vi "Save Date Yields.vi"(8 "error in (no error)":errorcluster, 10 "Cluster":T1, 11 "Master in":refnum<class "Master.lvclass">) -> (0 "error out":errorcluster, 3 "Master out":refnum<class "Master.lvclass">)   [LabVIEW 2014, in "Master.lvclass"]
uses:
  Master/Master.lvclass
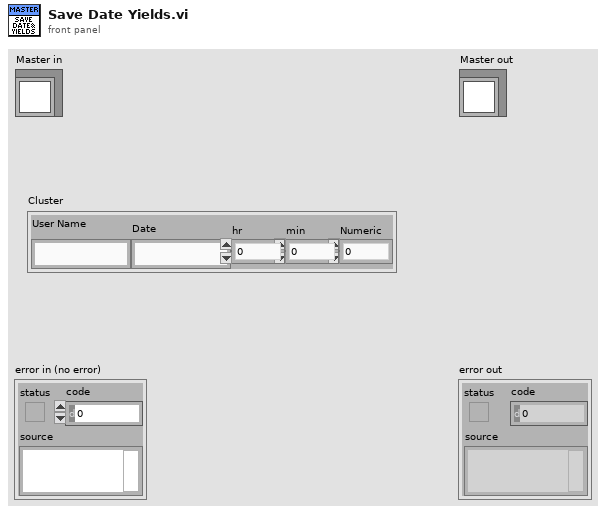
[diagram p1: front panel]
types:
  T1 = cluster{"User Name":string, "Date":string, "Numeric":dbl, "min":dbl, "hr":dbl}
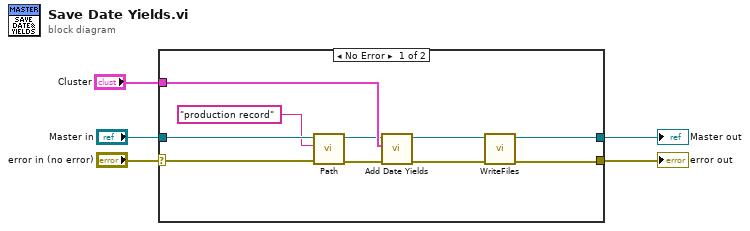
[diagram p0: block diagram]
diagram:
  n1 = case shown="No Error" "error in (no error)" {
    selector: "error in (no error)" -> [w14 w17]
    tunnel: [w11 w17] -> w4
    tunnel: [w12 w16] -> w2
    tunnel: "Master in" -> [w15 w16]
    tunnel: "Cluster" -> [w10 _]
    frame No Error {
      n2 = call-dynamic "Path.vi"("error in (no error)"=w14, "pathname"="production record", "Master in"=w15) -> ("error out"=w8:errorcluster, "Master out"=w9:refnum<class "Master.lvclass">)  [unwired: 7 in]
      n3 = call-dynamic "Add Date Yields.vi"("error in (no error)"=w8, "Cluster"=w10, "Master in"=w9) -> ("error out"=w6:errorcluster, "Master out"=w7:refnum<class "Master.lvclass">)  [unwired: 7 in]
      n4 = call-dynamic "WriteFiles.vi"("error in (no error)"=w6, "Master in"=w7) -> ("error out"=w11:errorcluster, "Master out"=w12:refnum<class "Master.lvclass">)  [unwired: 8 in]
    }
    frame Error {
    }
  }
  "error out" <- w4
  "Master out" <- w2
